vi "Construct.vi"(6 "File Change Map":T1 {"File Change Info"."Timestamp" format="%<%.0X %x>T"}, 7 "Bulk Attachments? (T)":bool=TRUE, 8 "error in (no error)":errorcluster {"code" format="Error %.0f"}, 9 "Working Directory":path, 10 "Top Page ID":string, 11 "Confluence":refnum<class "Confluence.lvclass">) -> (0 "error out":errorcluster {"code" format="Error %.0f"}, 3 "VIDoc Printer - Confluence Out":refnum<class "VIDoc Printer - Confluence.lvclass">)   [LabVIEW 2023, in "VIDoc Printer - Confluence.lvlib" / "VIDoc Printer - Confluence.lvclass"]
doc: "Confluence input is optional. Otherwise loads connection from Settings file."
uses:
  VIDoc Printer - Confluence.lvclass
  TypeDefs/File Change Map.ctl
  <userlib>/_PetranWay/LabVIEW Confluence API/Source/Confluence/Confluence Connection/Confluence.lvclass
  VIDoc Printer - Confluence.lvclass/VIDoc Printer - Confluence.ctl
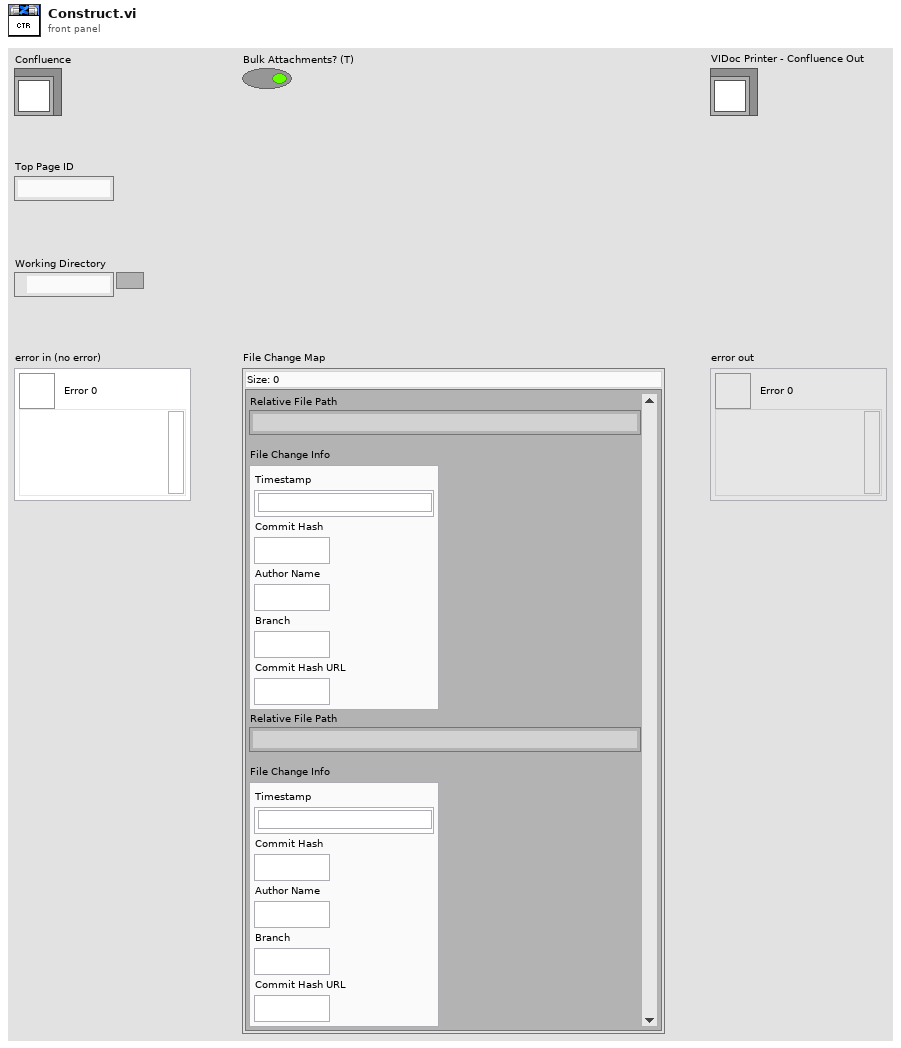
[diagram p1: front panel]
types:
  T1 = typedef "File Change Map.ctl" = map{string, cluster{"Timestamp":timestamp, "Commit Hash":string, "Author Name":string, "Branch":string, "Commit Hash URL":string}}
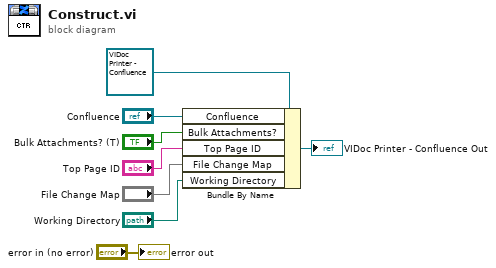
[diagram p0: block diagram]
diagram:
  n1 = Bundle By Name(cluster=refnum<class "VIDoc Printer - Confluence.lvclass"> refnum ("Confluence Printer out"), "Confluence"="Confluence", "Bulk Attachments?"="Bulk Attachments? (T)", "Top Page ID"="Top Page ID", "File Change Map"="File Change Map", "Working Directory"="Working Directory") -> (→"VIDoc Printer - Confluence Out":refnum<class "VIDoc Printer - Confluence.lvclass">)
  "error out" <- "error in (no error)"
